vi "Read All Samples.vi"(8 "error in (no error)":errorcluster, 11 "Stimulus in":refnum<class "Stimulus.lvclass">) -> (0 "error out":errorcluster, 2 "All Samples":dbl[](array[numeric]), 3 "Stimulus out":refnum<class "Stimulus.lvclass">)   [LabVIEW 2015, in "Stimulus.lvclass"]
uses:
  Stimulus.lvclass
  Stimulus.lvclass/Stimulus.ctl
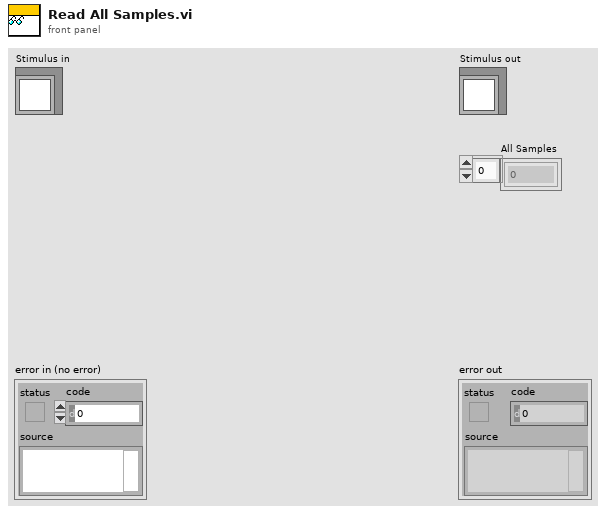
[diagram p1: front panel]
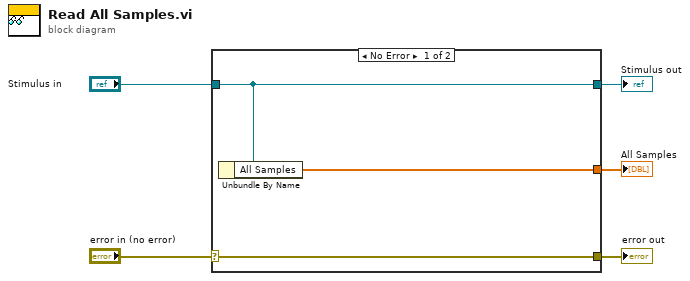
[diagram p0: block diagram]
diagram:
  n1 = case shown="No Error" "error in (no error)" {
    selector: "error in (no error)" -> [w8 w9]
    tunnel: [w8 w9] -> w4
    tunnel: [w7 w10] -> w2
    tunnel: "Stimulus in" -> [w7 w10]
    tunnel: [w6 _] -> w1
    frame No Error {
      n2 = Unbundle By Name(w7) -> ("All Samples"=w6:dbl[])
    }
    frame Error {
    }
  }
  "error out" <- w4
  "Stimulus out" <- w2
  "All Samples" <- w1
